vi "Create Process Events.vi"(8 "error in (no error)":errorcluster) -> (0 "error out":errorcluster, 2 "Process Events":T1)   [LabVIEW 2015, in "Simple Progress Bar.lvlib"]
uses:
  Simple Progress Bar.lvlib
  Process Events.ctl
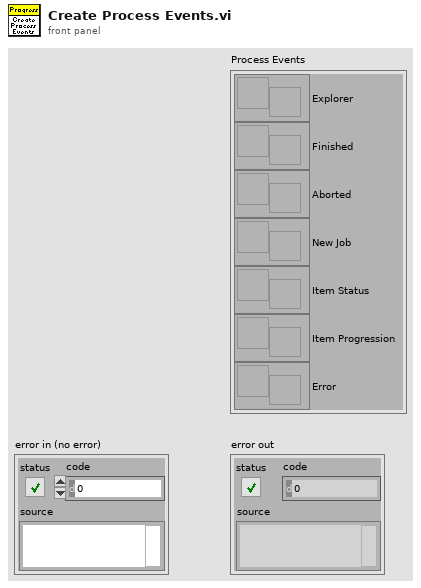
[diagram p1: front panel]
types:
  T1 = typedef "Simple Progress Bar.lvlib/Process Events.ctl" = cluster{"Explorer":refnum<user-event>, "Finished":refnum<user-event>, "Aborted":refnum<user-event>, "New Job":refnum<user-event>, "Item Status":refnum<user-event>, "Item Progression":refnum<user-event>, "Error":refnum<user-event>}
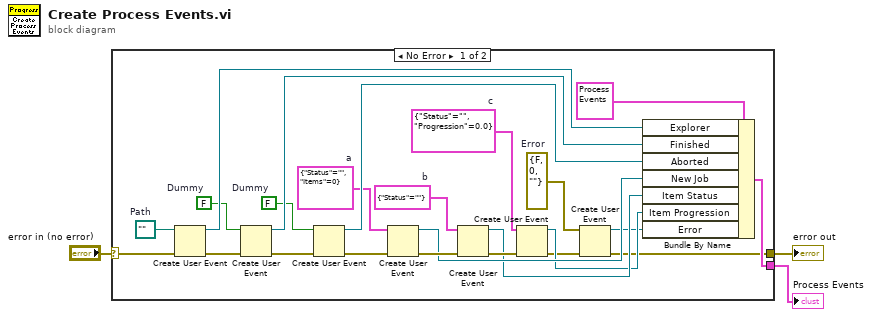
[diagram p0: block diagram]
diagram:
  n1 = case shown="No Error" "error in (no error)" {
    selector: "error in (no error)" -> [w26 w28]
    tunnel: [w6 w28] -> w2
    tunnel: [w27 _] -> w1
    frame No Error {
      w5 = errorcluster {"status"=FALSE, "code"=0, "source"=""}  # Error
      w13 = cluster{"Status":string, "Items":i32} {"Status"="", "Items"=0}  # a
      w12 = cluster{"Status":string} {"Status"=""}  # b
      w17 = path ""  # Path
      w19 = FALSE  # Dummy
      w20 = FALSE  # Dummy
      w11 = cluster{"Status":string, "Progression":dbl} {"Status"="", "Progression"=0.0}  # c
      n2 = Create User Event(user event datatype=w17, error in=w26) -> (user event=w25:refnum<user-event>, error out=w24:errorcluster)
      n3 = Create User Event(user event datatype=w20, error in=w24) -> (user event=w22:refnum<user-event>, error out=w23:errorcluster)
      n4 = Create User Event(user event datatype=w19, error in=w23) -> (user event=w21:refnum<user-event>, error out=w16:errorcluster)
      n5 = Create User Event(user event datatype=w13, error in=w16) -> (user event=w10:refnum<user-event>, error out=w15:errorcluster)
      n6 = Create User Event(user event datatype=w12, error in=w15) -> (user event=w9:refnum<user-event>, error out=w14:errorcluster)
      n7 = Create User Event(user event datatype=w11, error in=w14) -> (user event=w8:refnum<user-event>, error out=w7:errorcluster)
      n8 = Create User Event(user event datatype=w5, error in=w7) -> (user event=w4:refnum<user-event>, error out=w6:errorcluster)
      n9 = Bundle By Name(cluster=T1 {"Explorer"=refnum, "Finished"=refnum, "Aborted"=refnum, "New Job"=refnum, "Item Status"=refnum, "Item Progression"=refnum, "Error"=refnum} ("Process Events"), "Explorer"=w25, "Finished"=w22, "Aborted"=w21, "New Job"=w10, "Item Status"=w9, "Item Progression"=w8, "Error"=w4) -> (w27:T1)
    }
    frame Error {
    }
  }
  "error out" <- w2
  "Process Events" <- w1
